vi "Bus Status Count.vi"(8 "error in":errorcluster, 11 "Node Ptr":T1 format="%.0x") -> (0 "error out":errorcluster)   [LabVIEW 2020, in "AIM MIL-STD-1553 System Explorer.lvlib" / "Implementation.lvlib"]
uses:
  Implementation.lvlib
  <vilib>/NI VeriStand/Custom Device API/Custom Device Item Ref.ctl
  <vilib>/NI VeriStand/Custom Device API/Custom Device API.lvlib
panel:
  in  "General Header":cluster{"Section Name":string}={"Section Name"="MIL-STD-1553 - Bus Status Count"}
  in  "Description":string
  out "Name":string
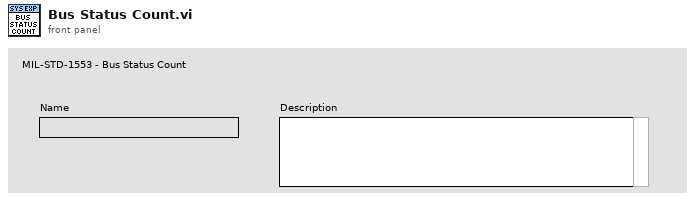
[diagram p1: front panel]
types:
  T1 = typedef "Custom Device API.lvlib/Custom Device Item Ref.ctl" = u64
  T2 = typedef "Custom Device API.lvlib/Custom Device Item Info.ctl" = cluster{"Name":string, "Is Channel":bool, "GUID":string, "Is Waveform":bool}
  T3 = typedef "Custom Device API.lvlib/Custom Device Commands.ctl" = enum16{"Default", "Item renamed", "Shutdown", "Dynamic button pressed"}
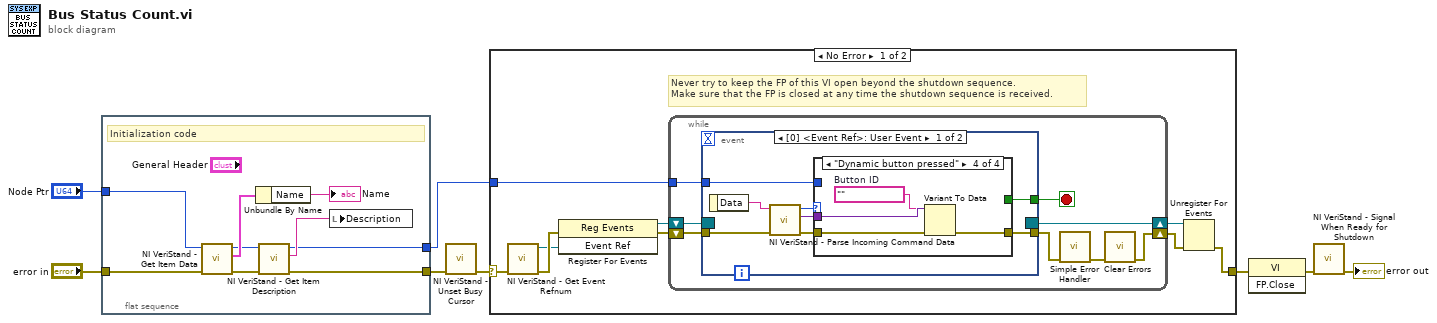
[diagram p0: block diagram]
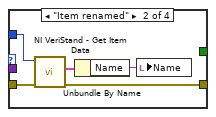
[diagram p3: hidden frame]
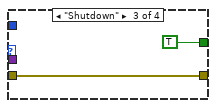
[diagram p4: hidden frame]
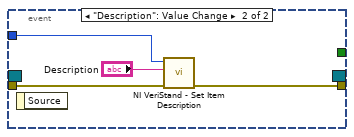
[diagram p5: hidden frame]
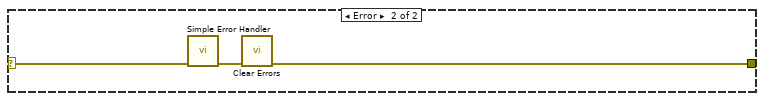
[diagram p6: hidden frame]
diagram:
  n1 = flat-sequence "Initialization code" {
    tunnel: "error in" -> [w9]
    tunnel: "Node Ptr" -> [w14]
    tunnel: [w10] -> w4
    tunnel: [w11] -> w1
    frame #0 {
      # "Initialization code"
      n2 = call <vilib>:"NI VeriStand - Get Item Data.vi"("error in (no error)"=w9, "Item Ref in"=w14) -> ("error out"=w12:errorcluster, "Item Info"=w17:T2, "Item Ref out"=w13:T1)  [unwired: 7 out]
      n3 = Unbundle By Name(w17) -> ("Name"=→"Name":string)
      n4 = call <vilib>:"NI VeriStand - Get Item Description.vi"("error in (no error)"=w12, "Item Ref in"=w13) -> ("error out"=w10:errorcluster, "Description"=w16:string, "Item Ref out"=w11:T1)  [unwired: 7 out]
      n5 = local write "Description"(w16) -> ()
    }
  }
  n6 = call <vilib>:"NI VeriStand - Unset Busy Cursor.vi"("error in (no error)"=w4) -> ("error out"=w3:errorcluster)  [unwired: 10 out]
  n7 = case shown="No Error" w3 {
    selector: w3 -> [w18 w61]
    tunnel: [w23 w59] -> w8
    tunnel: w1 -> [w19 _]
    frame No Error {
      # "Never try to keep the FP of this VI open beyond the shutdown sequence.\nMake sure that the FP is closed at any time the shutdown sequence is received."
      n8 = call <vilib>:"NI VeriStand - Get Event Refnum.vi"("error in (no error)"=w18) -> ("error out"=w26:errorcluster, "Event Ref"=w22:refnum<user-event>)  [unwired: 9 out]
      n9 = register-events(error in=w26, w22) -> (reference out=w20:refnum<event-registration>, error out=w21:errorcluster)  [unwired: 1 in]
      n10 = while {
        tunnel: w19 -> [w30]
        shift-right: [w27] -> w24
        shift-left: w21 -> [w33]
        shift-right: [w34] -> w25
        shift-left: w20 -> [w32]
        stop <- w31 stop-if-true
        n11 = event shown="[0] <Event Ref>: User Event" {
          selector: w32 -> [_ _]
          dyn-events: [_ _] -> w34
          timeout: _ -> [_ _]
          tunnel: w33 -> [w42 w57]
          tunnel: [w39 _] -> w31
          tunnel: [w38 w56] -> w29
          tunnel: w30 -> [w37 w58]
          event User Event {
            n12 = event-data() -> ("Data"=w35:string)  [unwired: 1 out]
            n13 = call <vilib>:"NI VeriStand - Parse Incoming Command Data.vi"("error in (no error)"=w42, "Incoming data"=w35) -> ("error out"=w41:errorcluster, "Outgoing data"=w36:variant, "Action"=w40:T3)  [unwired: 7 out]
            n14 = case shown="\"Dynamic button pressed\"" w40 {
              tunnel: w41 -> [w43 w48 w49 w54]
              tunnel: [_ _ TRUE _] -> w39
              tunnel: [w43 w45 w49 w51] -> w38
              tunnel: w37 -> [_ w47 _ _]
              tunnel: w36 -> [_ _ _ w53]
              frame Default {
              }
              frame "Item renamed" {
                n15 = call <vilib>:"NI VeriStand - Get Item Data.vi"("error in (no error)"=w48, "Item Ref in"=w47) -> ("error out"=w45:errorcluster, "Item Info"=w46:T2)  [unwired: 8 out]
                n16 = Unbundle By Name(w46) -> ("Name"=w44:string)
                n17 = local write "Name"(w44) -> ()
              }
              frame "Shutdown" {
              }
              frame "Dynamic button pressed" {
                w52 = ""  # Button ID
                n18 = Variant To Data(error in=w54, type=w52, Variant=w53) -> (error out=w51:errorcluster)  [unwired: 1 out]
              }
            }
          }
          event "Description": Value Change {
            n19 = event-data() -> ()  [unwired: 2 out]
            n20 = call <vilib>:"NI VeriStand - Set Item Description.vi"("error in (no error)"=w57, "Description"="Description", "Item Ref in"=w58) -> ("error out"=w56:errorcluster)  [unwired: 8 out]
          }
        }
        n21 = call <vilib>:"Simple Error Handler.vi"("error in (no error)"=w29) -> ("error out"=w28:errorcluster)  [unwired: 1 in, 7 out]
        n22 = call <vilib>:"Clear Errors.vi"("error in (no error)"=w28) -> ("error out"=w27:errorcluster)  [unwired: 1 in, 5 out]
      }
      n23 = Unregister For Events(event registration refnum=w25, error in=w24) -> (error out=w23:errorcluster)
    }
    frame Error {
      n24 = call <vilib>:"Simple Error Handler.vi"("error in (no error)"=w61) -> ("error out"=w60:errorcluster)  [unwired: 1 in, 7 out]
      n25 = call <vilib>:"Clear Errors.vi"("error in (no error)"=w60) -> ("error out"=w59:errorcluster)  [unwired: 1 in, 5 out]
    }
  }
  n26 = invoke on="Invoke Node" class="VI" method="FP.Close"(error in=w8) -> (error out=w7:errorcluster)  [unwired: 2 in, 2 out]
  n27 = call <vilib>:"NI VeriStand - Signal When Ready for Shutdown.vi"("error in (no error)"=w7) -> ("error out"=→"error out":errorcluster)  [unwired: 10 out]
